vi "InitilalizeTcpRaw.vi"(6 "恢复出厂":bool, 7 "仪器ID":string, 8 "错误输入（无错误）":errorcluster, 9 "VI引用":refnum<vi>, 10 "接口类型":u16(ring)=1 items=["GPIB"=1, "VXI"=2, "GPIB-VXI"=3, "Serial"=4, "PXI"=5, "TCPIP"=6, "USB"=7, "FireWire"=9], 11 "VISA资源名称":refnum<visa-resource-name>) -> (0 "错误输出":errorcluster, 2 "初始化成功?":bool, 3 "VISA资源名称输出":refnum<visa-resource-name>)   [LabVIEW 2018]
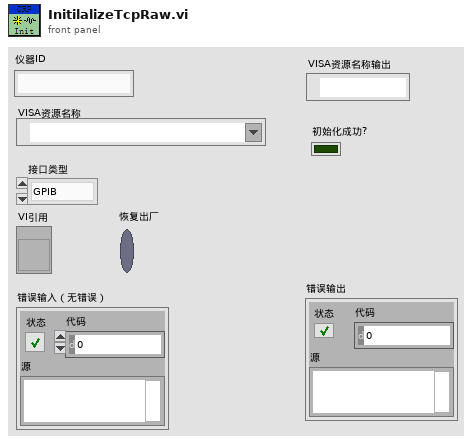
[diagram p1: front panel]
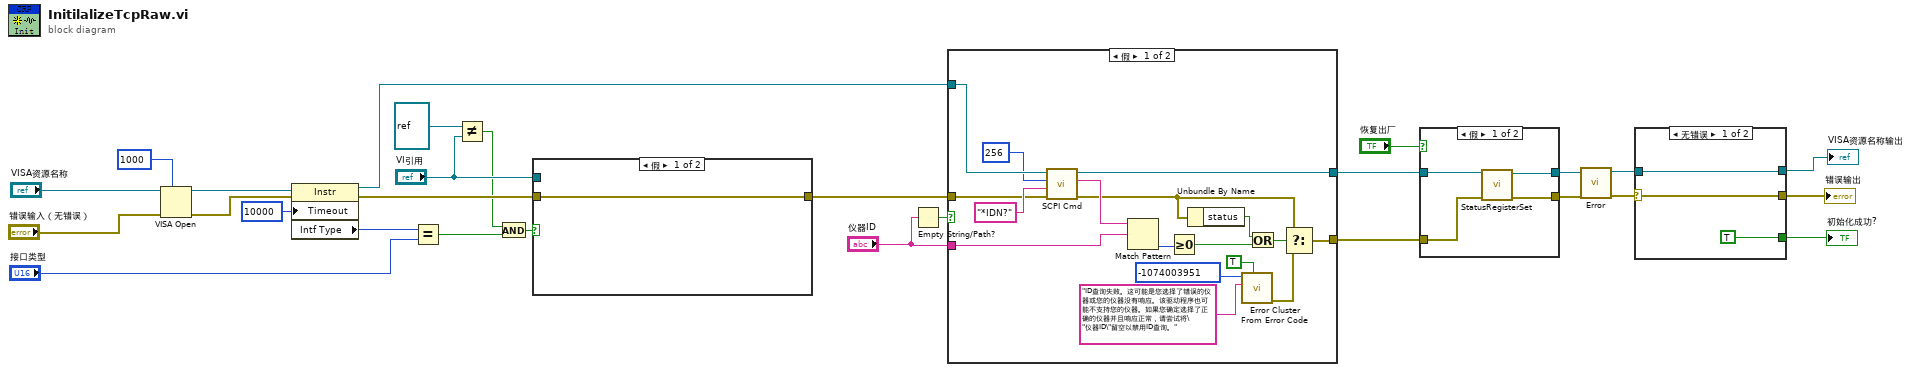
[diagram p0: block diagram]
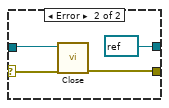
[diagram p2: hidden frame]
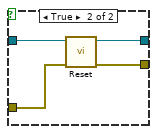
[diagram p3: hidden frame]
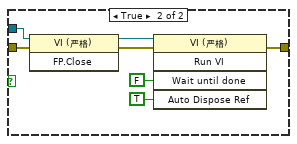
[diagram p5: hidden frame]
diagram:
  n1 = VISA Open(timeout (0)=u32 1000 ("VISA打开超时（0）"), error in (no error)="错误输入（无错误）", VISA resource name="VISA资源名称") -> (VISA resource name=w7:refnum<visa-resource-name>, error out=w6:errorcluster)  [unwired: 2 in]
  n2 = property class="Instr"(reference=w7, error in=w6, "Timeout"=u32 10000 ("General Settings:Timeout Value")) -> (reference out=w8:refnum<visa-resource-name>, error out=w22:errorcluster, "Intf Type"=w23:u16)
  n3 = Equal?(x=w23, y="接口类型") -> (x = y?=w10:bool)
  n4 = Not Equal?(x=refnum<vi> refnum ("VI引用"), y="VI引用") -> (x != y?=w5:bool)
  n5 = And(x=w5, y=w10) -> (x .and. y?=w11:bool)
  n6 = case shown="假" w11 {
    tunnel: w22 -> [w29 w35]
    tunnel: [w29 w31] -> w4
    tunnel: "VI引用" -> [_ w30]
    frame False {
    }
    frame True {
      n7 = invoke class="VI (严格)" method="FP.Close"(reference=w30, error in=w35) -> (reference out=w36:refnum<vi>, error out=w34:errorcluster)  [unwired: 1 in, 1 out]
      n8 = invoke class="VI (严格)" method="Run VI"(reference=w36, error in=w34, "Wait until done"=FALSE ("结束前等待"), "Auto Dispose Ref"=TRUE ("自动销毁引用")) -> (error out=w31:errorcluster)  [unwired: 1 in, 4 out]
    }
  }
  n9 = Empty String/Path?(string/path="仪器ID") -> (empty?=w21:bool)
  n10 = case shown="假" w21 {
    tunnel: w8 -> [w44 w55]
    tunnel: [w43 w55] -> w17
    tunnel: "仪器ID" -> [w53 _]
    tunnel: w4 -> [w40 w54]
    tunnel: [w37 w54] -> w18
    frame False {
      n11 = call "SCPI Cmd.vi"("VISA资源名称"=w44, "缓存区大小"=u32 256, "SCPI字符串"="*IDN?" ("写入缓冲区"), "错误输入（无错误）"=w40) -> ("VISA资源名称输出"=w43:refnum<visa-resource-name>, "读取缓冲区"=w39:string, "错误输出"=w38:errorcluster)  [unwired: 3 in, 1 out]
      n12 = Match Pattern(string=w39, regular expression=w53) -> (offset past match=w52:i32)  [unwired: 1 in, 3 out]
      n13 = Greater Or Equal To 0?(x=w52) -> (x >= 0?=w46:bool)
      n14 = Unbundle By Name(w38) -> ("status"=w45:bool)
      n15 = call <vilib>:"Error Cluster From Error Code.vi"("show call chain? (False)"=TRUE, "error message (\"\")"="ID查询失败。这可能是您选择了错误的仪器或您的仪器没有响应。该驱动程序也可能不支持您的仪器。如果您确定选择了正确的仪器并且响应正常，请尝试将\"仪器ID\"留空以禁用ID查询。" ("Source (VI Name)"), "error code (0)"=-1074003951 ("Code")) -> ("error out"=w48:errorcluster)  [unwired: 6 in]
      n16 = Or(x=w45, y=w46) -> (x .or. y?=w47:bool)
      n17 = Select(t=w38, s=w47, f=w48) -> (s? t:f=w37:errorcluster)
    }
    frame True {
    }
  }
  n18 = case shown="假" "恢复出厂" {
    tunnel: w18 -> [w57 w62]
    tunnel: w17 -> [w59 w63]
    tunnel: [w58 w61] -> w16
    tunnel: [w56 w60] -> w15
    frame False {
      n19 = call "StatusRegisterSet.vi"("错误输入（无错误）"=w57, "VISA引用句柄输入"=w59) -> ("错误输出"=w56:errorcluster, "VISA引用句柄输出"=w58:refnum<visa-resource-name>)  [unwired: 8 in]
    }
    frame True {
      n20 = call "Reset.vi"("错误输入（无错误）"=w62, "VISA资源名称"=w63) -> ("错误输出"=w60:errorcluster, "VISA资源名称输出"=w61:refnum<visa-resource-name>)  [unwired: 8 in]
    }
  }
  n21 = call "Error.vi"("error in (no error)"=w15, "VISA资源名称"=w16) -> ("错误输出"=w14:errorcluster, "VISA引用句柄输出"=w13:refnum<visa-resource-name>)  [unwired: 6 in, 2 out]
  n22 = case shown="无错误" w14 {
    selector: w14 -> [w66 w68]
    tunnel: [w66 w67] -> w28
    tunnel: [w65 refnum<visa-resource-name> refnum ("VISA引用句柄输出")] -> w27
    tunnel: w13 -> [w65 w69]
    tunnel: [TRUE ("布尔") _] -> w2
    frame No Error {
    }
    frame Error {
      n23 = call "Close.vi"("error in (no error)"=w68, "VISA资源名称"=w69) -> ("错误输出"=w67:errorcluster)  [unwired: 9 in]
    }
  }
  "错误输出" <- w28
  "VISA资源名称输出" <- w27
  "初始化成功?" <- w2
